vi "ZCAN_FilterClear.vi"(0 "error in (no error)":errorcluster caption="错误输入（无错误）", 2 "can_index_handle":u32, 5 "can_index":u32) -> (14 "error out":errorcluster caption="错误输出", 16 "can_index_handle(out)":u32, 19 "can_index(out)":u32)   [LabVIEW 2018]
doc: "清除滤波表格"
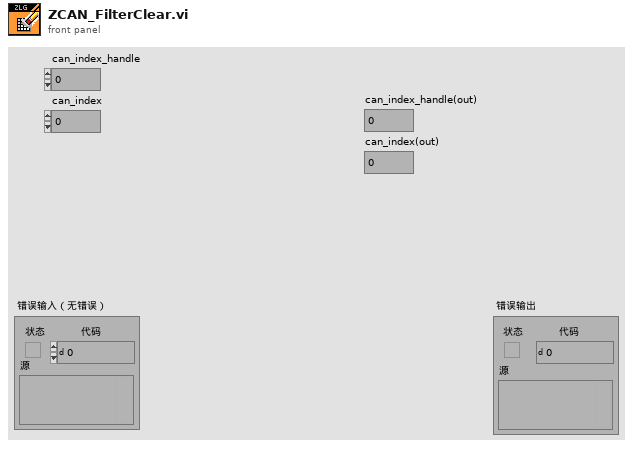
[diagram p1: front panel]
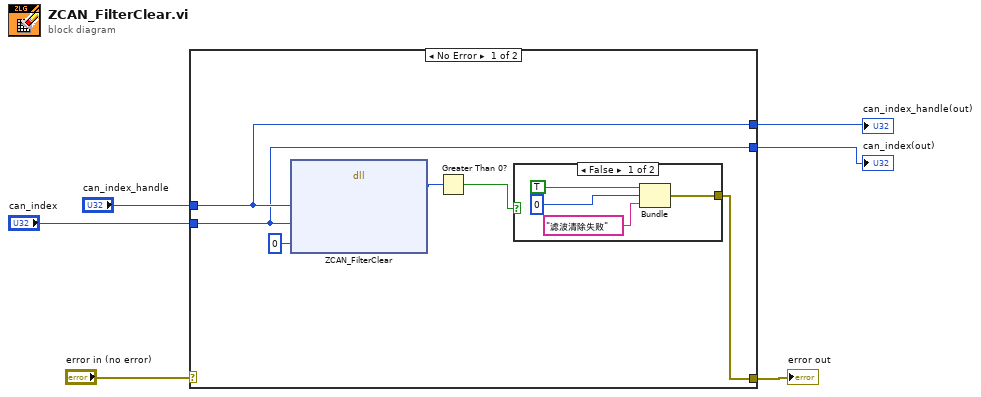
[diagram p0: block diagram]
diagram:
  n1 = case shown="No Error" "error in (no error)" {
    selector: "error in (no error)" -> [_ w17]
    tunnel: [w11 w17] -> w5
    tunnel: "can_index_handle" -> [w8 _]
    tunnel: "can_index" -> [w7 _]
    tunnel: [w8 _] -> w2
    tunnel: [w7 _] -> w1
    frame No Error {
      n2 = dll-call lib="PTH2\\abs CUsersadminDesktop以太网系列zlgcan_demo_CANET_TCPbinzlgcan_wrap.dll" fn="ZCAN_FilterClear"("device_handle"=w8, "can_index"=w7, "clear"=0) -> ("return"=w9:u32)  [unwired: 6 in, 2 out]
      n3 = Greater Than 0?(x=w9) -> (x > 0?=w12:bool)
      n4 = case shown="False" w12 {
        tunnel: [w13 _] -> w11
        frame False {
          n5 = Bundle("status"=TRUE, "code"=0, "消息"="滤波清除失败") -> (w13:cluster{"status":bool, "code":i32, "消息":string})  [unwired: 1 in]
        }
        frame True {
        }
      }
    }
    frame Error {
    }
  }
  "error out" <- w5
  "can_index_handle(out)" <- w2
  "can_index(out)" <- w1
